vi "LVClass_HasoSlopes ctor from MultiPupils Image.vi"(0 "HasoSlopes (const)":refnum<class "HasoSlopes.lvclass">, 5 "Image":refnum<class "Image.lvclass">, 7 "Haso configuration file":path, 9 "Start sub-aperture Array":T1[](array[typedef]), 11 "error in (no error)":errorcluster, 12 "check_calibration_checksum":bool) -> (4 "HasoSlopes (new)":refnum<class "HasoSlopes.lvclass">, 6 "Image (dup)":refnum<class "Image.lvclass">, 15 "error out":errorcluster)   [LabVIEW 2020, in "HasoSlopes.lvclass"]
uses:
  HasoSlopes.lvclass
  Image/Image.lvclass
  Controls/Point2D.ctl
  Controls/Handle creation.ctl
  HasoSlopes.lvclass/HasoSlopes.ctl
  Image/LVClass_Image Read Image.vi
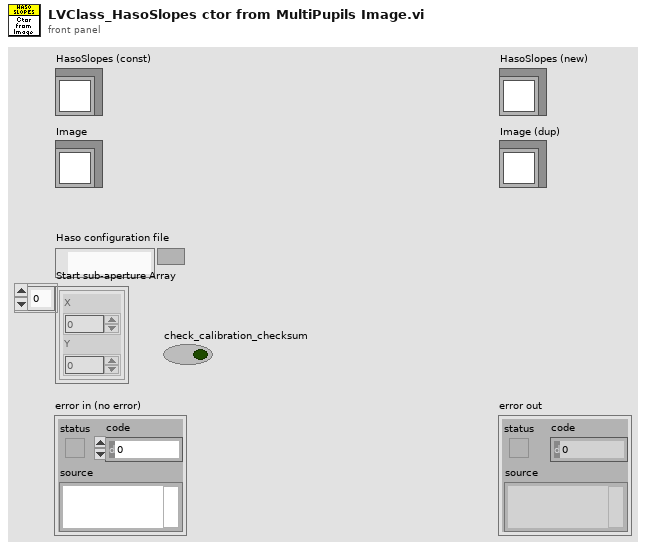
[diagram p1: front panel]
types:
  T1 = typedef "Point2D.ctl" = cluster{"X":u32, "Y":u32}
  T2 = typedef "Handle creation.ctl" = enum16{"By ctor", "By write function"}
  T3 = typedef "Struct_Image.ctl" = cluster{"Image_Handler":T4, "Number of bits":T5, "ImageSize":T1}
  T4 = typedef "ClassID.ctl" = i64
  T5 = typedef "Data alignment enum.ctl" = enum16{"8", "16", "32"}
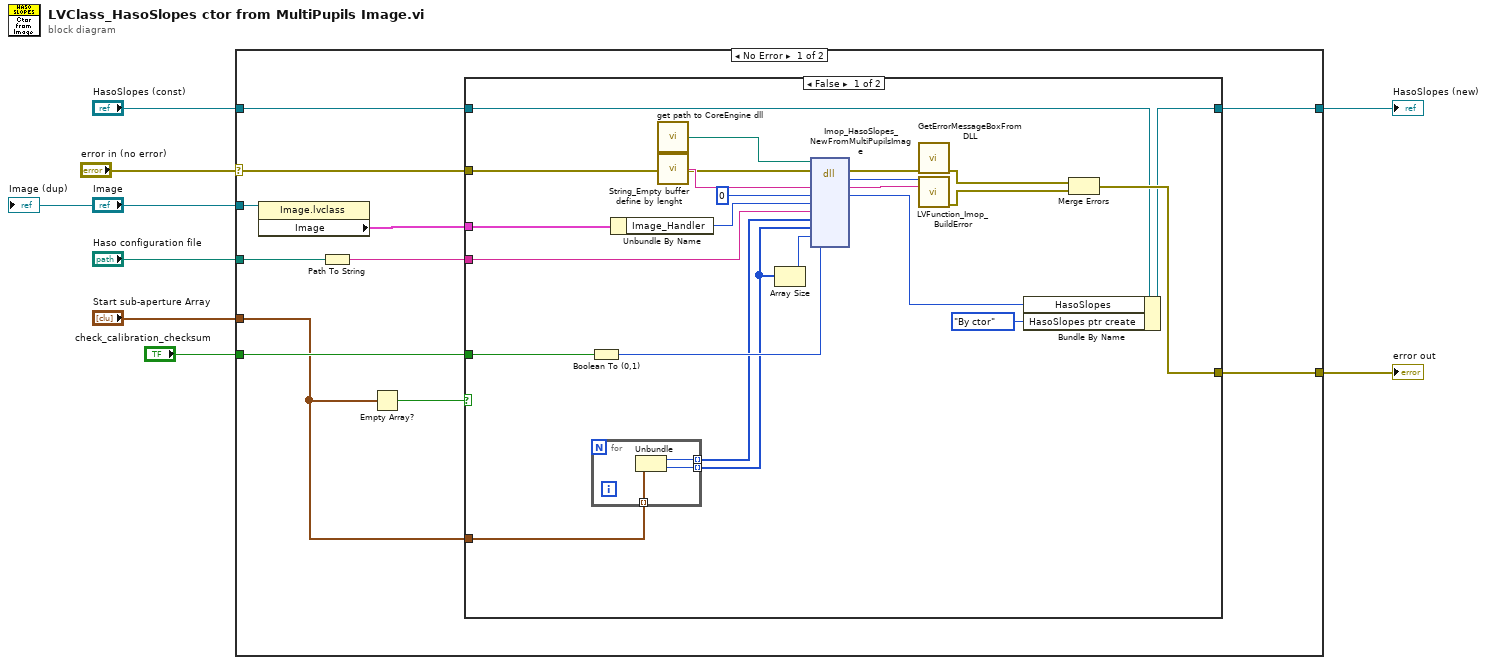
[diagram p0: block diagram]
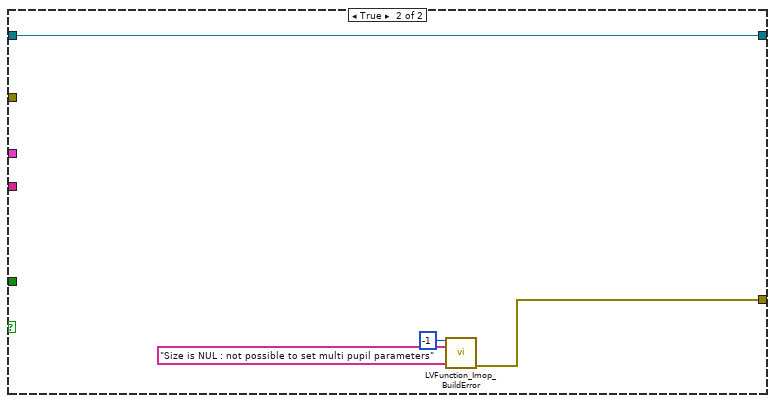
[diagram p2: hidden frame]
diagram:
  n1 = case shown="No Error" "error in (no error)" {
    selector: "error in (no error)" -> [w19 w51]
    tunnel: [w18 w51] -> w7
    tunnel: [w16 w50] -> w5
    tunnel: "HasoSlopes (const)" -> [w17 w50]
    tunnel: "Image" -> [w15 _]
    tunnel: "Haso configuration file" -> [w13 _]
    tunnel: "Start sub-aperture Array" -> [w10 _]
    tunnel: "check_calibration_checksum" -> [w11 _]
    frame No Error {
      n2 = property class="Image.lvclass"(reference=w15) -> ("Image"=w14:T3)  [unwired: 1 in, 2 out]
      n3 = Path To String(path=w13) -> (string=w12:string)
      n4 = Empty Array?(array=w10) -> (empty?=w9:bool)
      n5 = case shown="False" w9 {
        tunnel: w19 -> [w35 _]
        tunnel: [w34 w46] -> w18
        tunnel: w17 -> [w33 w49]
        tunnel: [w32 w49] -> w16
        tunnel: w14 -> [w29 _]
        tunnel: w12 -> [w27 _]
        tunnel: w11 -> [w24 _]
        tunnel: w10 -> [w23 _]
        frame False {
          n6 = Boolean To (0,1)(Boolean=w24) -> (0, 1=w25:i16)
          n7 = for {
            tunnel: w23 -> [w45] mode=indexing
            tunnel: [w44] -> w22 mode=indexing
            tunnel: [w43] -> w21 mode=indexing
            n8 = Unbundle(w45) -> ("X"=w44:u32, "Y"=w43:u32)
          }
          n9 = Unbundle By Name(w29) -> ("Image_Handler"=w28:T4)
          n10 = call "get path to CoreEngine dll.vi"() -> ("path to wavekit library"=w38:path)  [unwired: 14 in, 1 out]
          n11 = call "String_Empty buffer define by lenght.vi"() -> ("Empty buffer"=w39:string)  [unwired: 1 in]
          n12 = Array Size(array=w21) -> (size(s)=w20:i32)
          n13 = dll-call lib="D:/FLE/0.Code/CoreEngine4_Suite/LV2011_interface/DLLs/c_interface_vc100.dll" fn="Imop_HasoSlopes_NewFromMultiPupilsImage"(path in=w38, error in=w35, "Message"=w39, "HasoSlopes"=0, "Image"=w28, "HASO configuration path"=w27, "x_start_subpupil"=w22, "y_start_subpupil"=w21, "size"=w20, "check_calibration_checksum"=w25) -> (error out=w42:errorcluster, "return type"=w40:i32, "Message"=w41:string, "HasoSlopes"=w26:i64)  [unwired: 7 in, 1 out]
          n14 = call "GetErrorMessageBoxFromDLL.vi"("error IN"=w42) -> ("error OUT"=w37:errorcluster)  [unwired: 10 in]
          n15 = call "LVFunction_Imop_BuildError.vi"("code"=w40, "String to Prepend to source (\"\")"=w41) -> ("error out"=w36:errorcluster)  [unwired: 13 in]
          n16 = Bundle By Name(cluster=w33, "HasoSlopes"=w26, "HasoSlopes ptr create"=Handle_creation."By ctor") -> (w32:refnum<class "HasoSlopes.lvclass">)
          n17 = Merge Errors(w37, w36) -> (w34:errorcluster)
        }
        frame True {
          n18 = call "LVFunction_Imop_BuildError.vi"("code"=-1, "String to Prepend to source (\"\")"="Size is NUL : not possible to set multi pupil parameters" ("String to Prepend to source (\"\")")) -> ("error out"=w46:errorcluster)  [unwired: 13 in]
        }
      }
    }
    frame Error {
    }
  }
  "error out" <- w7
  "HasoSlopes (new)" <- w5
  "Image (dup)" <- "Image"
